vi "COMI WFM Get Cur Pos.vi"(10 "ch":i32, 11 "hDevice":u32) -> (2 "function return":i32, 3 "hDevice out":u32)   [LabVIEW 2017, in "Comidll.lvlib"]
doc: "long (COMI_WFM_GetCurPos) (HANDLE hDevice, int ch);"
uses:
  <userlib>/Comidll/Comidll.lvlib
  <userlib>/Comidll/Comidll.dll
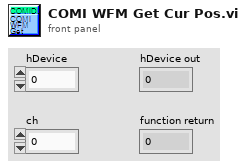
[diagram p1: front panel]
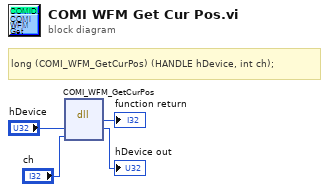
[diagram p0: block diagram]
diagram:
  # "long\t(COMI_WFM_GetCurPos) (HANDLE hDevice, int ch);"
  n1 = dll-call lib="C:/Program Files/National Instruments/LabVIEW 2017/user.lib/Comidll/Comidll.*" fn="COMI_WFM_GetCurPos"("hDevice"="hDevice", "ch"="ch") -> (→"function return":i32, "hDevice"=→"hDevice out":u32)  [unwired: 4 in, 2 out]
